vi "Configure Trigger (Setup & Hold).vi"(0 "VISA resource name":refnum<visa-resource-name>, 1 "Setup Time (4.0ns)":dbl=4e-09, 2 "Hold Time (4.0ns)":dbl=4e-09, 5 "Clock Edge (0: Rising)":u16(ring) items=["Rising", "Falling"], 7 "Clock Source (0: Channel 1)":u16(ring) items=["Channel 1"=0, "Channel 2"=1, "Channel 3"=2, "Channel 4"=3, "Aux"=12, "Digital Channel 0"=14, "Digital Channel 1"=15, "Digital Channel 2"=16, "Digital Channel 3"=17, "Digital Channel 4"=18, "Digital Channel 5"=19, "Digital Channel 6"=20, "Digital Channel 7"=21, "Digital Channel 8"=22, "Digital Channel 9"=23, "Digital Channel 10"=24, "Digital Channel 11"=25, "Digital Channel 12"=26, "Digital Channel 13"=27, "Digital Channel 14"=28, "Digital Channel 15"=29], 9 "Data Source (1: Channel 2)":u16(ring)=1 items=["Channel 1"=0, "Channel 2"=1, "Channel 3"=2, "Channel 4"=3, "Aux"=12, "Digital Channel 0"=14, "Digital Channel 1"=15, "Digital Channel 2"=16, "Digital Channel 3"=17, "Digital Channel 4"=18, "Digital Channel 5"=19, "Digital Channel 6"=20, "Digital Channel 7"=21, "Digital Channel 8"=22, "Digital Channel 9"=23, "Digital Channel 10"=24, "Digital Channel 11"=25, "Digital Channel 12"=26, "Digital Channel 13"=27, "Digital Channel 14"=28, "Digital Channel 15"=29], 11 "error in (no error)":errorcluster, 12 "Enable Multiple Data Sources (F: Disabled)":bool, 13 "Multiple Data Sources":u16[](array[ring]) items=["Channel 1"=0, "Channel 2"=1, "Channel 3"=2, "Channel 4"=3, "Aux"=12, "Digital Channel 0"=14, "Digital Channel 1"=15, "Digital Channel 2"=16, "Digital Channel 3"=17, "Digital Channel 4"=18, "Digital Channel 5"=19, "Digital Channel 6"=20, "Digital Channel 7"=21, "Digital Channel 8"=22, "Digital Channel 9"=23, "Digital Channel 10"=24, "Digital Channel 11"=25, "Digital Channel 12"=26, "Digital Channel 13"=27, "Digital Channel 14"=28, "Digital Channel 15"=29]) -> (4 "VISA resource name out":refnum<visa-resource-name>, 15 "error out":errorcluster)   [LabVIEW 2009, in "Tektronix DPO MSO 2000 4000 Series.lvlib"]
doc: "Configures sethold trigger settings for an oscilloscope. A sethold trigger occurs when a setup or hold violation happens."
uses:
  <instrlib>/Tektronix DPO MSO 2000 4000 Series/Tektronix DPO MSO 2000 4000 Series.lvlib
panel:
  # "MSO Only"
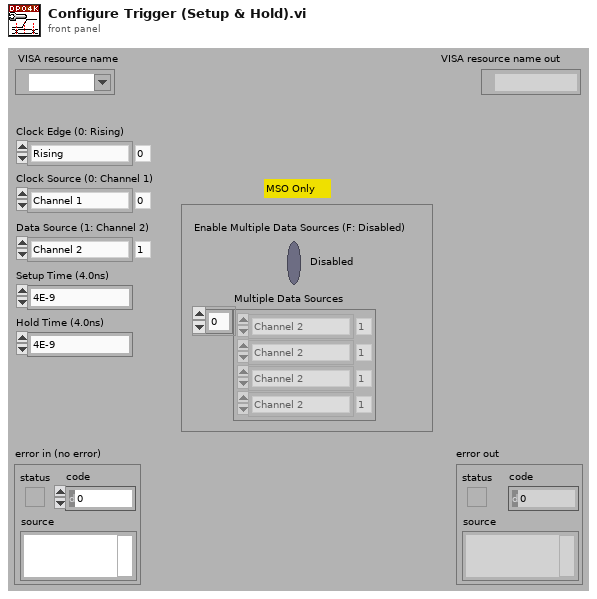
[diagram p1: front panel]
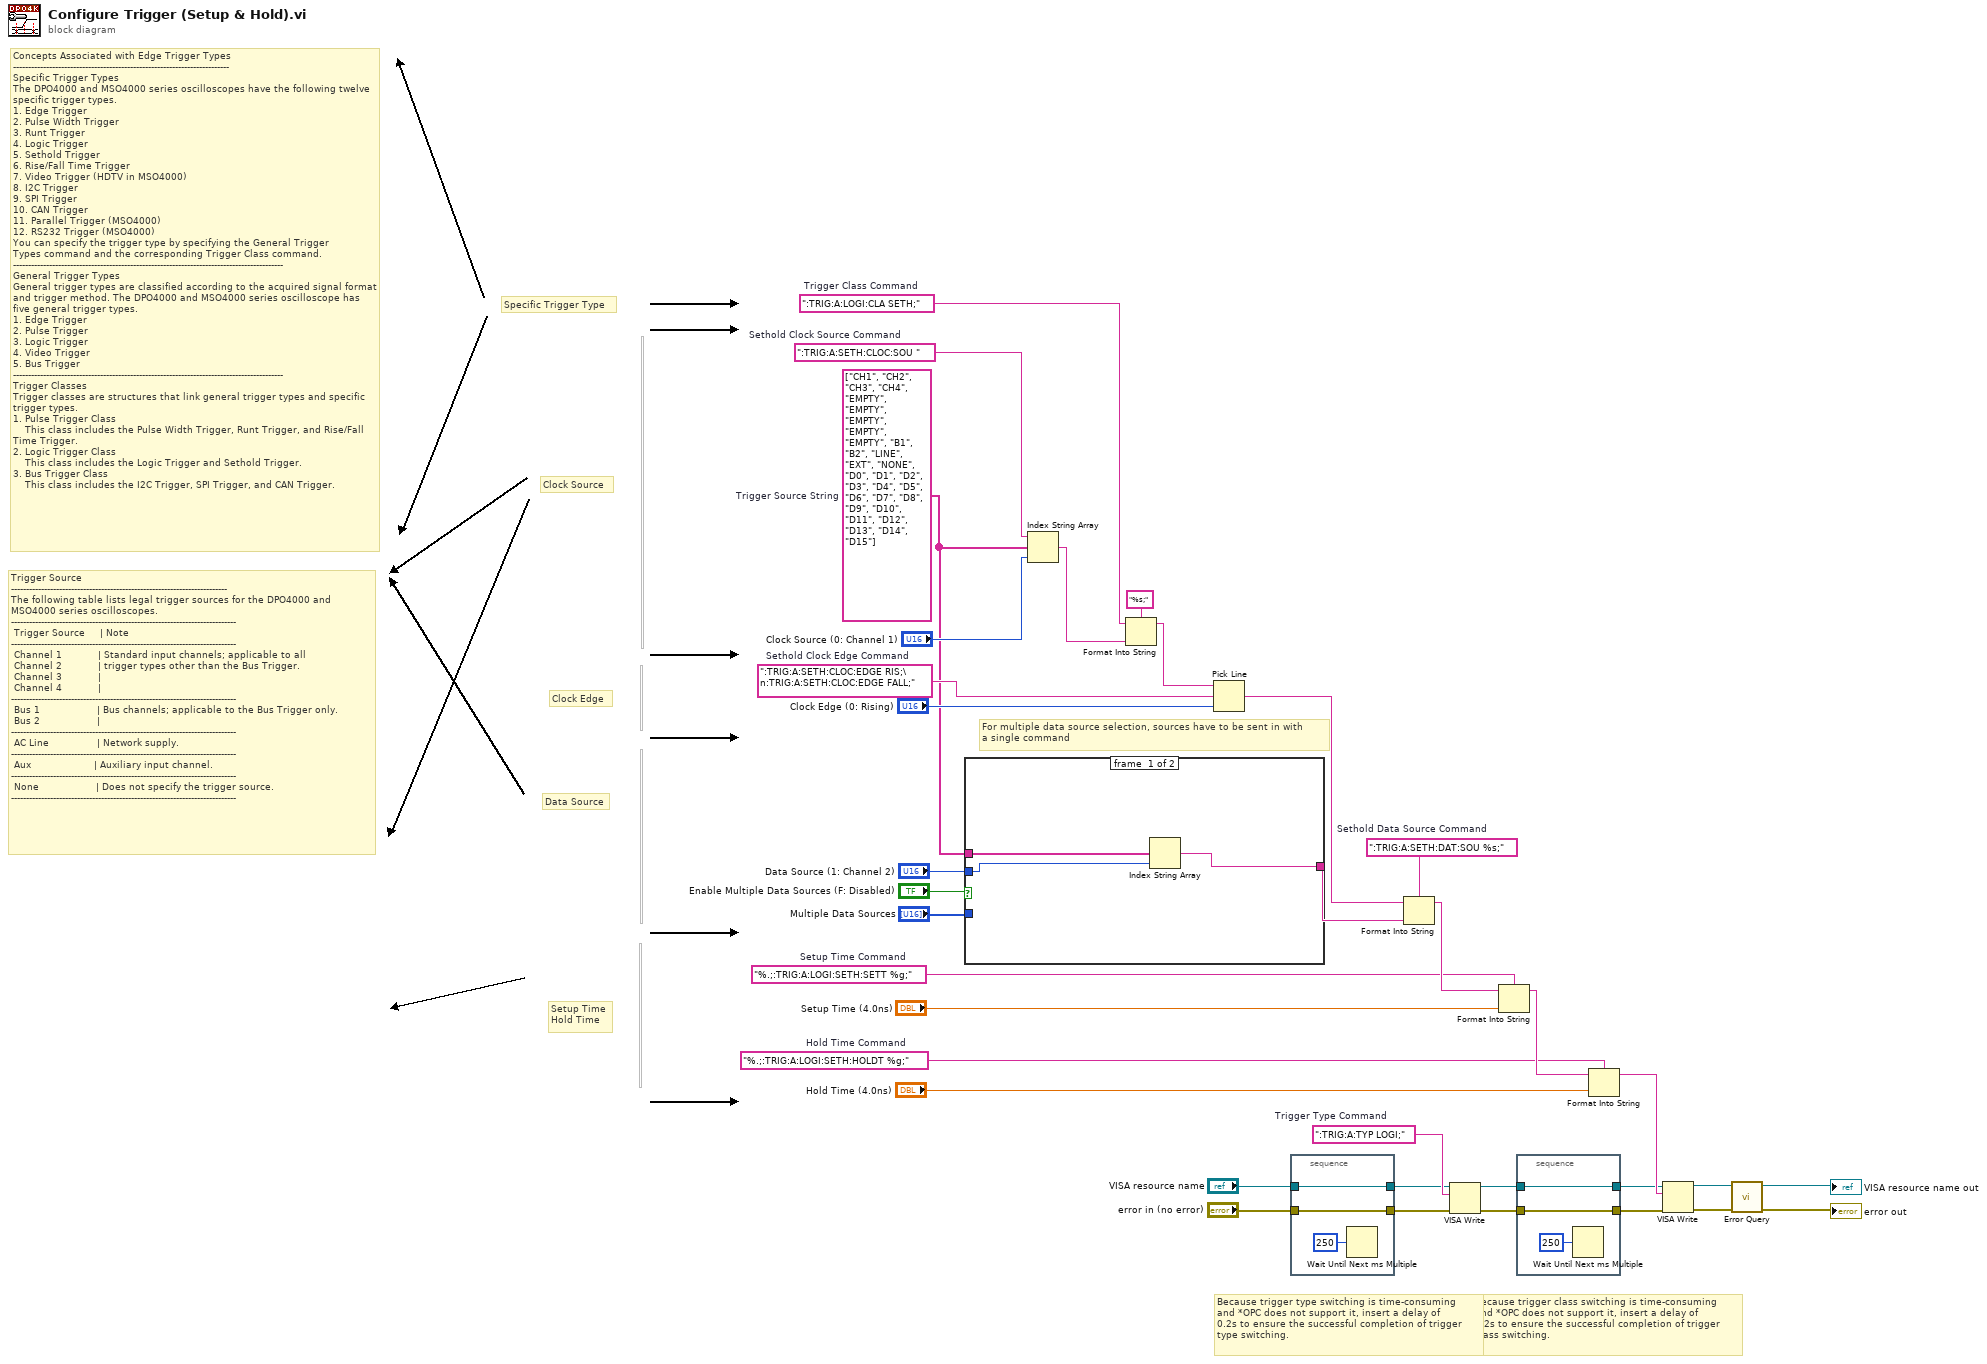
[diagram p0: block diagram]
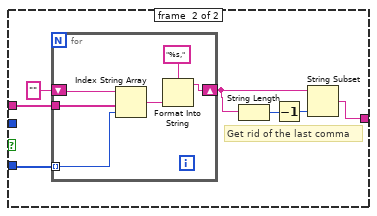
[diagram p2: hidden frame]
diagram:
  w1 = ":TRIG:A:SETH:DAT:SOU %s;"  # Sethold Data Source Command
  w4 = string[] ["CH1", "CH2", "CH3", "CH4", "EMPTY", "EMPTY", "EMPTY", "EMPTY", "EMPTY", "B1", "B2", "LINE", "EXT", "NONE", "D0", "D1", "D2", "D3", "D4", "D5", "D6", "D7", "D8", "D9", "D10", "D11", "D12", "D13", "D14", "D15"]  # Trigger Source String
  w22 = "%.;:TRIG:A:LOGI:SETH:HOLDT %g;"  # Hold Time Command
  w25 = "%.;:TRIG:A:LOGI:SETH:SETT %g;"  # Setup Time Command
  w18 = ":TRIG:A:SETH:CLOC:EDGE RIS;\n:TRIG:A:SETH:CLOC:EDGE FALL;"  # Sethold Clock Edge Command
  w20 = ":TRIG:A:LOGI:CLA SETH;"  # Trigger Class Command
  w34 = ":TRIG:A:TYP LOGI;"  # Trigger Type Command
  w35 = ":TRIG:A:SETH:CLOC:SOU "  # Sethold Clock Source Command
  # "For multiple data source selection, sources have to be sent in with\na single command"
  # "Trigger Source\n------------------------------------------------------------------------\nThe following table lists legal trigger sources for the DPO4000 and MSO4000 series oscilloscopes.\n---------------------------------------------------------------------------\n Trigger Source     | Note                                                           \n---------------------------------------------------------------------------\n Channel 1            | Standard input channels; applicable to all      \n Channel 2            | trigger types other than the Bus Trigger.         \n Channel 3            |     \n Channel 4            |\n---------------------------------------------------------------------------\n Bus 1                   | Bus channels; applicable to the Bus Trigger only.\n Bus 2                   | \n---------------------------------------------------------------------------\n AC Line                | Network supply.\n---------------------------------------------------------------------------\n Aux                     | Auxiliary input channel.\n---------------------------------------------------------------------------\n None                   | Does not specify the trigger source.\n---------------------------------------------------------------------------"
  # "Concepts Associated with Edge Trigger Types\n------------------------------------------------------------------------\nSpecific Trigger Types\nThe DPO4000 and MSO4000 series oscilloscopes have the following twelve specific trigger types.\n1. Edge Trigger\n2. Pulse Width Trigger\n3. Runt Trigger\n4. Logic Trigger\n5. Sethold Trigger\n6. Rise/Fall Time Trigger\n7. Video Trigger (HDTV in MSO4000)\n8. I2C Trigger\n9. SPI Trigger\n10. CAN Trigger\n11. Parallel Trigger (MSO4000)\n12. RS232 Trigger (MSO4000)\nYou can specify the trigger type by specifying the General Trigger \nTypes command and the corresponding Trigger Class command.\n------------------------------------------------------------------------------------------\nGeneral Trigger Types \nGeneral trigger types are classified according to the acquired signal format and trigger method. The DPO4000 and MSO4000 series oscilloscope has five general trigger types.\n1. Edge Trigger\n2. Pulse Trigger\n3. Logic Trigger\n4. Video Trigger\n5. Bus Trigger\n------------------------------------------------------------------------------------------\nTrigger Classes\nTrigger classes are structures that link general trigger types and specific trigger types.\n1. Pulse Trigger Class\n    This class includes the Pulse Width Trigger, Runt Trigger, and Rise/Fall Time Trigger.\n2. Logic Trigger Class\n    This class includes the Logic Trigger and Sethold Trigger.\n3. Bus Trigger Class\n    This class includes the I2C Trigger, SPI Trigger, and CAN Trigger."
  # "Because trigger class switching is time-consuming\nand *OPC does not support it, insert a delay of\n0.2s to ensure the successful completion of trigger\nclass switching."
  # "Because trigger type switching is time-consuming\nand *OPC does not support it, insert a delay of\n0.2s to ensure the successful completion of trigger\ntype switching."
  # "Setup Time\nHold Time"
  # "Data Source"
  # "Clock Edge"
  # "Clock Source"
  # "Specific Trigger Type"
  n1 = case shown="False" "Enable Multiple Data Sources (F: Disabled)" {
    tunnel: "Data Source (1: Channel 2)" -> [w37 _]
    tunnel: w4 -> [w38 w44]
    tunnel: "Multiple Data Sources" -> [_ w45]
    tunnel: [w36 w42] -> w2
    frame #0 {
      n2 = Index String Array(1:w37, 2:w38) -> (0:w36:string)  [unwired: 1 in]
    }
    frame #1 {
      # "Get rid of the last comma"
      n3 = for {
        tunnel: w45 -> [w49] mode=indexing
        tunnel: w44 -> [w50]
        shift-right: [w47] -> w41
        shift-left: "" -> [w51]
        n4 = Index String Array(1:w49, 2:w50, 3:w51) -> (0:w48:string)
        n5 = Format Into String(format string="%s,", w48) -> (resulting string=w47:string)  [unwired: 2 in, 1 out]
      }
      n6 = String Length(string=w41) -> (length=w40:i32)
      n7 = Decrement(x=w40) -> (x-1=w39:i32)
      n8 = String Subset(string=w41, length (rest)=w39) -> (substring=w42:string)  [unwired: 1 in]
    }
  }
  n9 = Index String Array(1:"Clock Source (0: Channel 1)", 2:w4, 3:w35) -> (0:w28:string)
  n10 = Format Into String(format string="%s;", initial string=w20, w28) -> (resulting string=w19:string)  [unwired: 1 in, 1 out]
  n11 = Pick Line(string ("")=w19, multi-line string=w18, line index="Clock Edge (0: Rising)") -> (output string=w16:string)
  n12 = stacked-sequence {
    tunnel: "VISA resource name" -> [w53]
    tunnel: [w53] -> w33
    tunnel: "error in (no error)" -> [w52]
    tunnel: [w52] -> w32
    frame #0 {
      n13 = Wait Until Next ms Multiple(millisecond multiple=u32 250) -> ()  [unwired: 1 out]
    }
  }
  n14 = Format Into String(format string=w1, initial string=w16, w2) -> (resulting string=w26:string)  [unwired: 1 in, 1 out]
  n15 = VISA Write(VISA resource name=w33, write buffer=w34, error in (no error)=w32) -> (VISA resource name out=w31:refnum<visa-resource-name>, error out=w30:errorcluster)  [unwired: 1 out]
  n16 = Format Into String(format string=w25, initial string=w26, "Setup Time (4.0ns)") -> (resulting string=w23:string)  [unwired: 1 in, 1 out]
  n17 = stacked-sequence {
    tunnel: w31 -> [w56]
    tunnel: [w56] -> w12
    tunnel: w30 -> [w55]
    tunnel: [w55] -> w11
    frame #0 {
      n18 = Wait Until Next ms Multiple(millisecond multiple=u32 250) -> ()  [unwired: 1 out]
    }
  }
  n19 = Format Into String(format string=w22, initial string=w23, "Hold Time (4.0ns)") -> (resulting string=w15:string)  [unwired: 1 in, 1 out]
  n20 = VISA Write(VISA resource name=w12, write buffer=w15, error in (no error)=w11) -> (VISA resource name out=w10:refnum<visa-resource-name>, error out=w9:errorcluster)  [unwired: 1 out]
  n21 = call <instrlib>:"Error Query.vi"("error in (no error)"=w9, "VISA resource name"=w10) -> ("error out"=→"error out":errorcluster, "VISA resource name out"=→"VISA resource name out":refnum<visa-resource-name>)  [unwired: 6 in, 2 out]
